vi "mod_Generate Integer Interpolation Filter.vi"(11 "interpolation factor":i32=1) -> (1 "filter coefficients out":dbl[](graph), 2 "total length":i32, 3 "polyphase filter out (2D)":dbl[][](array[numeric]), 5 "polyphase filter out (1D)":dbl[](array[numeric]))   [LabVIEW 2020, in "niAMT.lvlib"]
uses:
  <vilib>/addons/Modulation/niAMT.lvlib
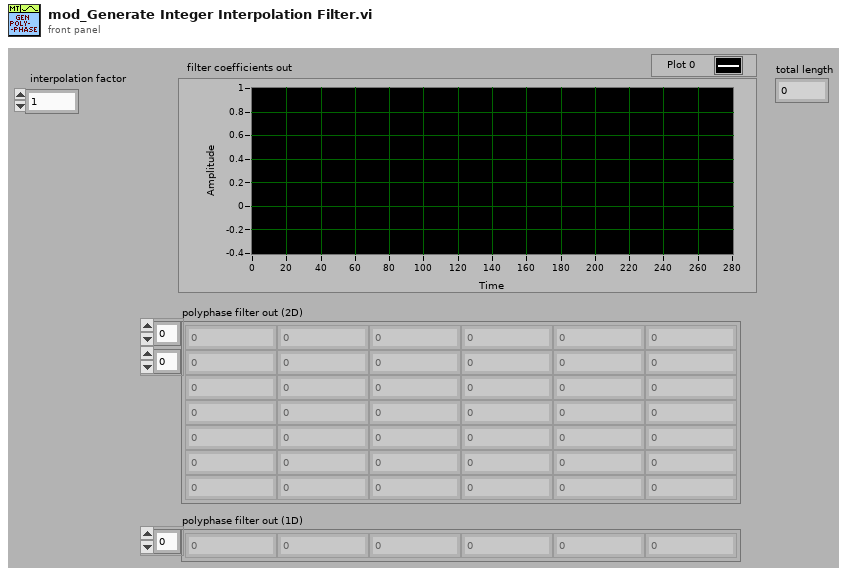
[diagram p1: front panel]
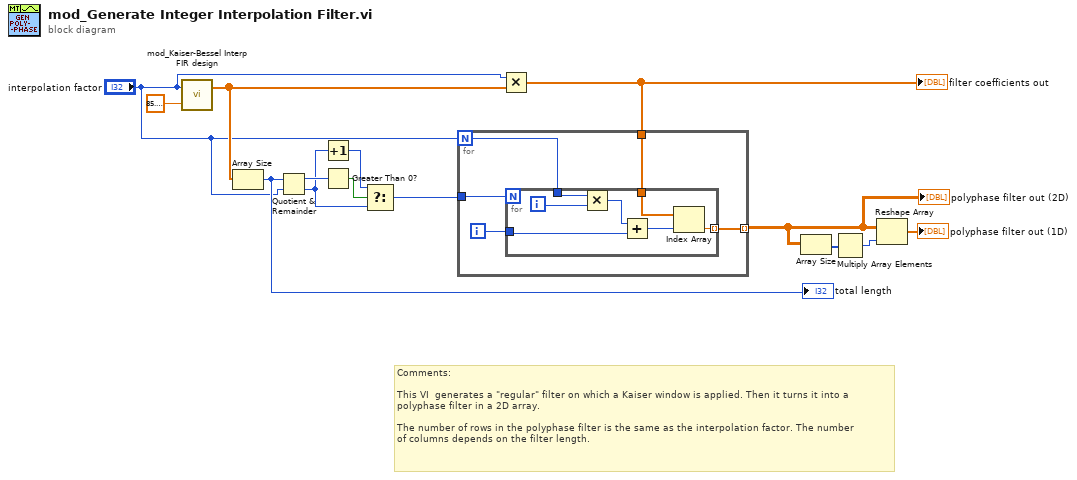
[diagram p0: block diagram]
diagram:
  # "Comments:\n\nThis VI  generates a \"regular\" filter on which a Kaiser window is applied. Then it turns it into a\npolyphase filter in a 2D array.\n\nThe number of rows in the polyphase filter is the same as the interpolation factor. The number\nof columns depends on the filter length."
  n1 = call <vilib>:"mod_Kaiser-Bessel Interp FIR design.vi"("Stop Attenuation"=85.00000000000051, "interpolation factor"="interpolation factor") -> ("h"=w2:dbl[])  [unwired: 1 out]
  n2 = Array Size(array=w2) -> (size(s)=w4:i32)
  "total length" <- w4
  n3 = Quotient & Remainder(x=w4, y="interpolation factor") -> (x-y*floor(x/y)=w12:i32, floor(x/y)=w11:i32)
  n4 = Increment(x=w11) -> (x+1=w10:i32)
  n5 = Greater Than 0?(x=w12) -> (x > 0?=w13:bool)
  n6 = Select(t=w10, s=w13, f=w11) -> (s? t:f=w9:i32)
  n7 = Multiply(x="interpolation factor", y=w2) -> (x*y=w3:dbl[])
  "filter coefficients out" <- w3
  n8 = for {
    N: "interpolation factor" -> [w17]
    tunnel: w9 -> [w19]
    tunnel: w3 -> [w16]
    tunnel: [w15] -> w5 mode=indexing
    i -> [w18]
    n9 = for {
      N: w19 -> [_]
      tunnel: w18 -> [w23]
      tunnel: w17 -> [w25]
      tunnel: w16 -> [w21]
      tunnel: [w20] -> w15 mode=indexing
      i -> [w26]
      n10 = Multiply(x=w25, y=w26) -> (x*y=w24:i32)
      n11 = Add(x=w24, y=w23) -> (x+y=w22:i32)
      n12 = Index Array(array=w21, index=w22) -> (element=w20:dbl)
    }
  }
  "polyphase filter out (2D)" <- w5
  n13 = Array Size(array=w5) -> (size(s)=w7:i32[])
  n14 = Multiply Array Elements(1:w7) -> (0:w8:i32)
  n15 = Reshape Array(w5, w8) -> (→"polyphase filter out (1D)":dbl[])
